vi "relayOpenCircuitTest.vi"() -> ()   [LabVIEW 2023]
panel:
  in  "switchTime/s":i32=50
  in  "relay 2 (unshort)":bool
  in  "flag 2":bool
  out "error out":errorcluster
  in  "relay 1 (open)":bool
  in  "flag 1":bool
  in  "error in (no error)":errorcluster
  in  "VISA relay":refnum<visa-resource-name>
  in  "VISA 2110 current":refnum<visa-resource-name>="USB0::0x05E6::0x2110::8017058::INSTR"
  in  "VISA 2110 voltage":refnum<visa-resource-name>="USB0::0x05E6::0x2110::8016020::INSTR"
  out "error out 4":errorcluster
  out "error out 3":errorcluster
  in  "stop 5":bool
  out "Current through 330 ohm resistor inner segment/mA 6":cluster{"Y":dbl[], "Y":dbl[]}[](graph)
  out "Voltage across 330 ohm resistor 7":dbl[](graph)
  out "Voltage across 330 ohm resistor 8":dbl[](array[numeric])
  out "Current time":timestamp
  out "Voltage/V":cluster{"Y":dbl[], "Y":dbl[]}[](graph)
  out "Voltage":dbl[](graph)
  out "Voltage":dbl[](array[numeric])
  in  "Filename 4":path caption="Filename"
  in  "Camera":bool=TRUE
  out "Start time":timestamp
  in  "Countdown/s":i32=3
  out "Timer":dbl
  in  "error in (no error) 3":errorcluster
  in  "error in (no error) 2":errorcluster
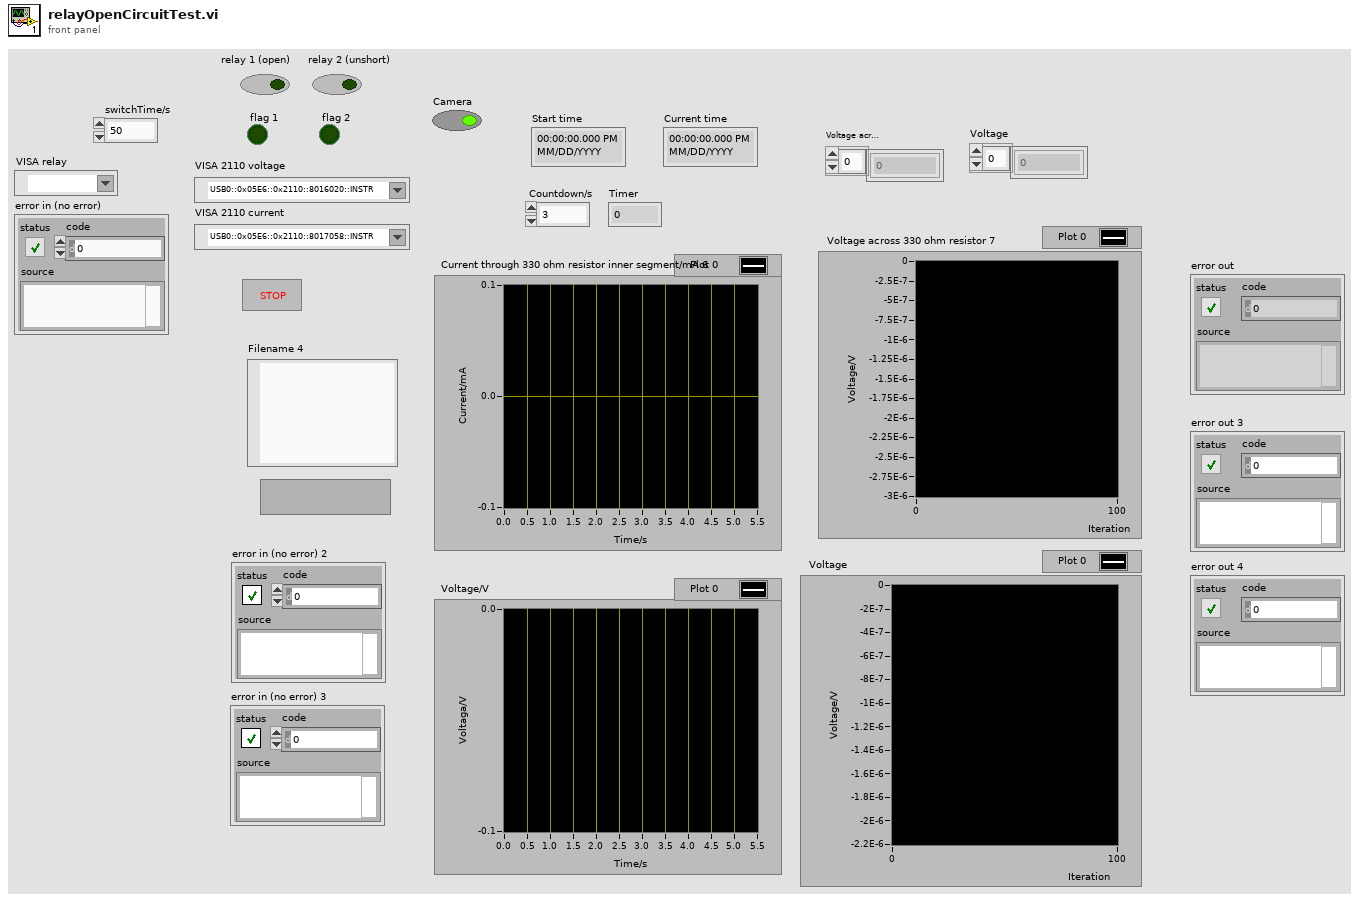
[diagram p1: front panel]
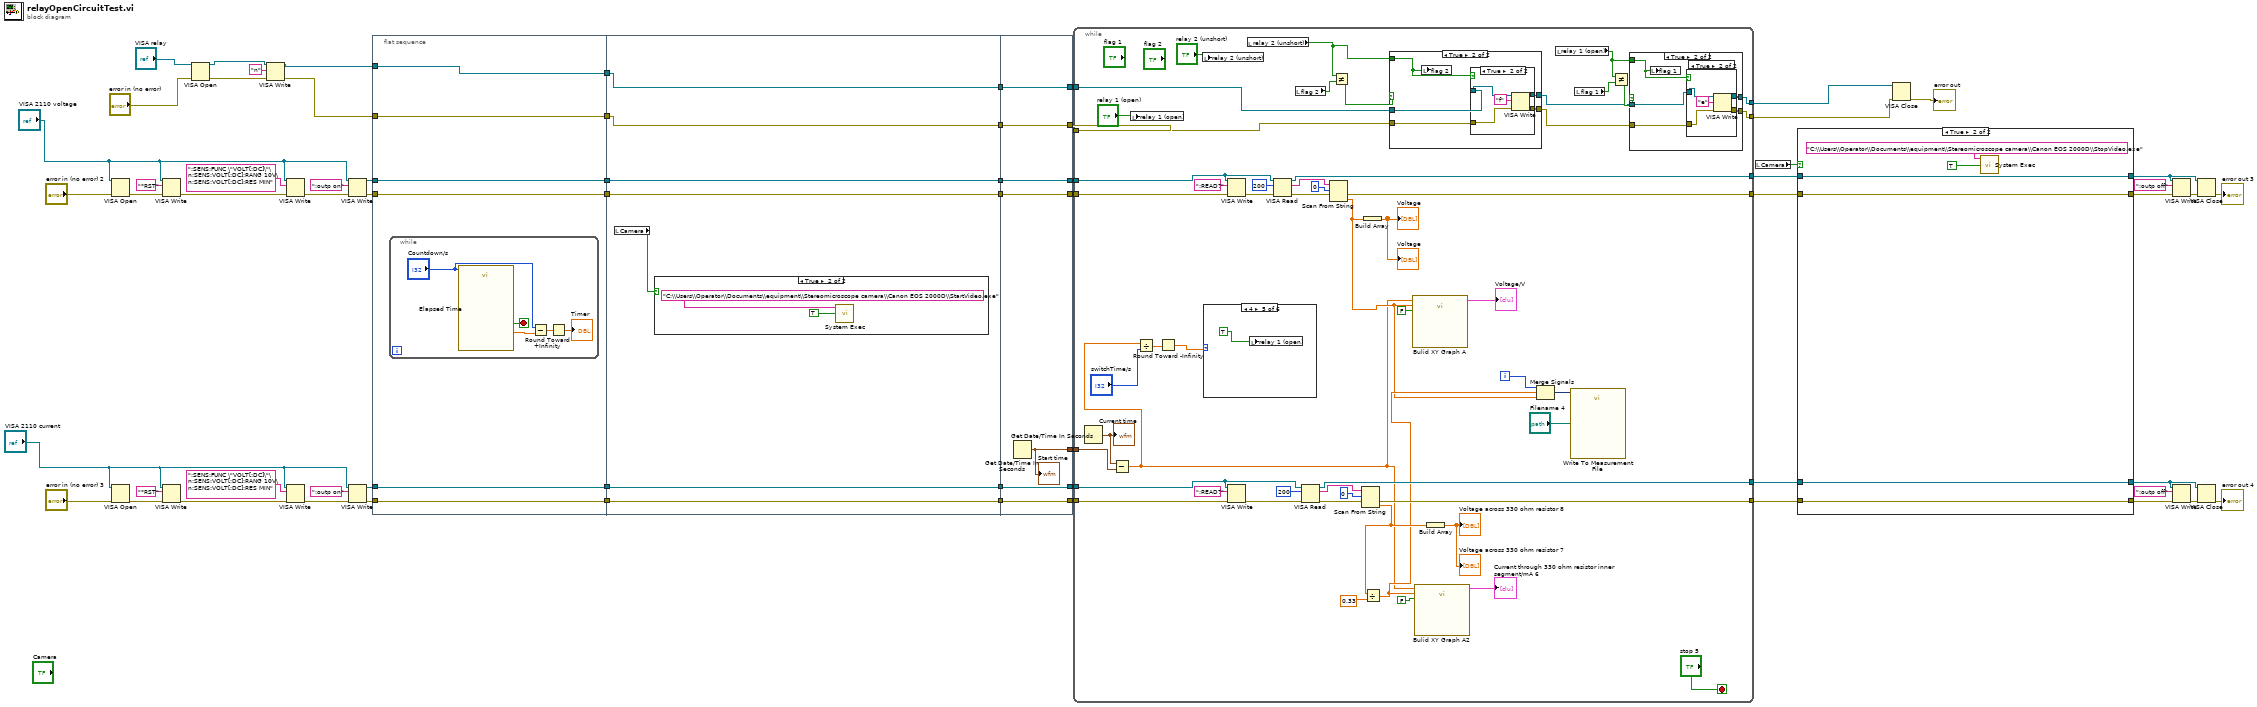
[diagram p0: block diagram]
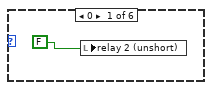
[diagram p3: hidden frame]
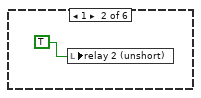
[diagram p4: hidden frame]
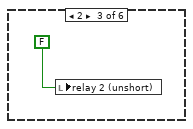
[diagram p5: hidden frame]
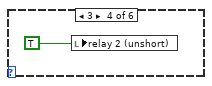
[diagram p6: hidden frame]
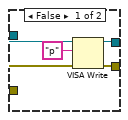
[diagram p9: hidden frame]
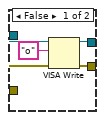
[diagram p11: hidden frame]
diagram:
  n1 = VISA Open(error in (no error)="error in (no error) 2", VISA resource name="VISA 2110 voltage") -> (error out=w64:errorcluster)  [unwired: 3 in, 1 out]
  n2 = VISA Open(error in (no error)="error in (no error) 3", VISA resource name="VISA 2110 current") -> (error out=w58:errorcluster)  [unwired: 3 in, 1 out]
  n3 = VISA Write(VISA resource name="VISA 2110 voltage", write buffer="*RST" ("数据"), error in (no error)=w64) -> (error out=w63:errorcluster)  [unwired: 2 out]
  n4 = VISA Write(VISA resource name="VISA 2110 current", write buffer="*RST" ("数据"), error in (no error)=w58) -> (error out=w57:errorcluster)  [unwired: 2 out]
  n5 = VISA Open(error in (no error)="error in (no error)", VISA resource name="VISA relay") -> (VISA resource name=w4:refnum<visa-resource-name>, error out=w3:errorcluster)  [unwired: 3 in]
  n6 = VISA Write(VISA resource name=w4, write buffer="n", error in (no error)=w3) -> (VISA resource name out=w1:refnum<visa-resource-name>, error out=w2:errorcluster)  [unwired: 1 out]
  n7 = VISA Write(VISA resource name="VISA 2110 voltage", write buffer=":SENS:FUNC \"VOLT[:DC]\"\n:SENS:VOLT[:DC]:RANG 10V\n:SENS:VOLT[:DC]:RES MIN" ("address string"), error in (no error)=w63) -> (error out=w62:errorcluster)  [unwired: 2 out]
  n8 = VISA Write(VISA resource name="VISA 2110 current", write buffer=":SENS:FUNC \"VOLT[:DC]\"\n:SENS:VOLT[:DC]:RANG 10V\n:SENS:VOLT[:DC]:RES MIN" ("address string"), error in (no error)=w57) -> (error out=w56:errorcluster)  [unwired: 2 out]
  n9 = VISA Write(VISA resource name="VISA 2110 voltage", write buffer=":outp on" ("数据"), error in (no error)=w62) -> (VISA resource name out=w42:refnum<visa-resource-name>, error out=w41:errorcluster)  [unwired: 1 out]
  n10 = VISA Write(VISA resource name="VISA 2110 current", write buffer=":outp on" ("数据"), error in (no error)=w56) -> (VISA resource name out=w40:refnum<visa-resource-name>, error out=w39:errorcluster)  [unwired: 1 out]
  n11 = flat-sequence {
    tunnel: w41 -> [w69]
    tunnel: w42 -> [w70]
    tunnel: [w70] -> w50
    tunnel: [w69] -> w49
    tunnel: w40 -> [w68]
    tunnel: [w68] -> w48
    tunnel: w39 -> [w67]
    tunnel: [w67] -> w47
    tunnel: [w66] -> w14
    tunnel: w1 -> [w66]
    tunnel: [w65] -> w11
    tunnel: w2 -> [w65]
    tunnel: w50 -> [w82]
    tunnel: w49 -> [w81]
    tunnel: [w82] -> w46
    tunnel: [w81] -> w45
    tunnel: [w79] -> w44
    tunnel: w48 -> [w79]
    tunnel: [w78] -> w43
    tunnel: w47 -> [w78]
    tunnel: w14 -> [w77]
    tunnel: [w77] -> w13
    tunnel: w11 -> [w76]
    tunnel: [w76] -> w10
    tunnel: [w89] -> w38
    tunnel: [w90] -> w36
    tunnel: [w91] -> w37
    tunnel: w46 -> [w91]
    tunnel: w45 -> [w90]
    tunnel: [w88] -> w35
    tunnel: w44 -> [w88]
    tunnel: [w87] -> w34
    tunnel: w43 -> [w87]
    tunnel: [w86] -> w12
    tunnel: w13 -> [w86]
    tunnel: [w85] -> w9
    tunnel: w10 -> [w85]
    frame #0 {
      n12 = while {
        stop <- w73 stop-if-true
        n13 = call "Elapsed Time"("Time Target (s)"="Countdown/s") -> ("Elapsed Time (s)"=w75:dbl, "Time has Elapsed"=w73:bool)  [unwired: 11 in, 6 out]
        n14 = Subtract(x="Countdown/s", y=w75) -> (x-y=w72:dbl)
        n15 = Round Toward +Infinity(x=w72) -> (ceil(x): smallest int >= x=→"Timer":dbl)
      }
    }
    frame #1 {
      n16 = local read "Camera"() -> (w80:bool)
      n17 = case shown="True" w80 {
        frame False {
        }
        frame True {
          n18 = call <vilib>:"System Exec.vi"("wait until completion? (T)"=TRUE, "command line"="C:\\Users\\Operator\\Documents\\equipment\\Stereomicroscope camera\\Canon EOS 2000D\\StartVideo.exe") -> ()  [unwired: 6 in, 4 out]
        }
      }
    }
    frame #2 {
      n19 = Get Date/Time In Seconds() -> (seconds since 1Jan1904=w89:timestamp)
      "Start time" <- w89
    }
  }
  n20 = while {
    tunnel: w38 -> [w145]
    tunnel: w37 -> [w144]
    tunnel: w36 -> [w143]
    tunnel: w35 -> [w142]
    tunnel: w34 -> [w141]
    tunnel: [w139] -> w26
    tunnel: [w138] -> w24
    tunnel: [w137] -> w22
    tunnel: [w136] -> w20
    tunnel: w12 -> [w125]
    tunnel: w9 -> [w128]
    tunnel: [w132] -> w8
    tunnel: [w131] -> w7
    i -> [w135]
    stop <- "stop 5" stop-if-true
    n21 = Get Date/Time In Seconds() -> (seconds since 1Jan1904=w107:timestamp)
    "Current time" <- w107
    n22 = Subtract(x=w107, y=w145) -> (x-y=w95:dbl)
    n23 = local write "relay 1 (open)"("relay 1 (open)") -> ()
    n24 = Divide(x=w95, y="switchTime/s") -> (x/y=w96:dbl)
    n25 = Round Toward -Infinity(1:w96) -> (0:w94:dbl)
    n26 = local write "relay 2 (unshort)"("relay 2 (unshort)") -> ()
    n27 = case shown="4" w94 {
      frame 0 {
        n28 = local write "relay 2 (unshort)"(FALSE) -> ()
      }
      frame 1 {
        n29 = local write "relay 2 (unshort)"(TRUE) -> ()
      }
      frame 2 {
        n30 = local write "relay 2 (unshort)"(FALSE) -> ()
      }
      frame 3 {
        n31 = local write "relay 2 (unshort)"(TRUE) -> ()
      }
      frame 4 {
        n32 = local write "relay 1 (open)"(TRUE) -> ()
      }
      frame 5, Default {
      }
    }
    n33 = VISA Write(VISA resource name=w144, write buffer=":READ?" ("数据"), error in (no error)=w143) -> (error out=w120:errorcluster)  [unwired: 2 out]
    n34 = VISA Write(VISA resource name=w142, write buffer=":READ?" ("数据"), error in (no error)=w141) -> (error out=w111:errorcluster)  [unwired: 2 out]
    n35 = local read "relay 2 (unshort)"() -> (w92:bool)
    n36 = VISA Read(VISA resource name=w144, byte count=200 ("字节总数"), error in (no error)=w120) -> (VISA resource name out=w139:refnum<visa-resource-name>, read buffer=w122:string, error out=w121:errorcluster)  [unwired: 1 out]
    n37 = local read "flag 2"() -> (w130:bool)
    n38 = VISA Read(VISA resource name=w142, byte count=200 ("字节总数"), error in (no error)=w111) -> (VISA resource name out=w137:refnum<visa-resource-name>, read buffer=w113:string, error out=w112:errorcluster)  [unwired: 1 out]
    n39 = Scan From String(input string=w122, initial scan location=u32 0 ("初始扫描位置"), error in=w121) -> (error out=w138:errorcluster, output 1=w100:dbl)  [unwired: 2 in, 2 out]
    n40 = Not Equal?(x=w92, y=w130) -> (x != y?=w129:bool)
    n41 = Scan From String(input string=w113, initial scan location=u32 0 ("初始扫描位置"), error in=w112) -> (error out=w136:errorcluster, output 1=w102:dbl)  [unwired: 2 in, 2 out]
    n42 = Build Array(w100) -> (→"Voltage" →"Voltage":dbl[])
    n43 = Divide(x=w102, y=0.33) -> (x/y=w101:dbl)
    n44 = case shown="True" w129 {
      tunnel: w92 -> [_ w157]
      tunnel: w128 -> [w152 w153]
      tunnel: [w151 w156] -> w127
      tunnel: [w152 w155] -> w126
      tunnel: w125 -> [w151 w154]
      frame False {
      }
      frame True {
        n45 = local write "flag 2"(w157) -> ()
        n46 = case shown="True" w157 {
          tunnel: w154 -> [w159 w167]
          tunnel: w153 -> [w158 w165]
          tunnel: [w161 w164] -> w156
          tunnel: [w160 w163] -> w155
          frame False {
            n47 = VISA Write(VISA resource name=w159, write buffer="p", error in (no error)=w158) -> (VISA resource name out=w161:refnum<visa-resource-name>, error out=w160:errorcluster)  [unwired: 1 out]
          }
          frame True {
            n48 = VISA Write(VISA resource name=w167, write buffer="f", error in (no error)=w165) -> (VISA resource name out=w164:refnum<visa-resource-name>, error out=w163:errorcluster)  [unwired: 1 out]
          }
        }
      }
    }
    n49 = call "Bulid XY Graph A"("Reset"=FALSE, "Y Input"=w100, "X Input"=w95) -> ("XY Graph"=→"Voltage/V":cluster{"X":dbl[], "Y":dbl[]}[])  [unwired: 7 in, 1 out]
    n50 = call "Bulid XY Graph A2"("Reset"=FALSE, "Y Input"=w101, "X Input"=w95) -> ("XY Graph"=→"Current through 330 ohm resistor inner segment/mA 6":cluster{"X":dbl[], "Y":dbl[]}[])  [unwired: 7 in, 1 out]
    n51 = Build Array(w102) -> (→"Voltage across 330 ohm resistor 8" →"Voltage across 330 ohm resistor 7":dbl[])
    n52 = Merge Signals(w135, w101, w100) -> (w124:dynamicdata)
    n53 = local read "relay 1 (open)"() -> (w98:bool)
    n54 = call "Write To Measurement File"("Signals"=w124, "Filename"="Filename 4") -> ()  [unwired: 15 in, 3 out]
    n55 = local read "flag 1"() -> (w134:bool)
    n56 = Not Equal?(x=w98, y=w134) -> (x != y?=w133:bool)
    n57 = case shown="True" w133 {
      tunnel: w98 -> [_ w174]
      tunnel: w126 -> [w169 w170]
      tunnel: [w168 w173] -> w132
      tunnel: [w169 w172] -> w131
      tunnel: w127 -> [w168 w171]
      frame False {
      }
      frame True {
        n58 = local write "flag 1"(w174) -> ()
        n59 = case shown="True" w174 {
          tunnel: w171 -> [w176 w184]
          tunnel: w170 -> [w175 w182]
          tunnel: [w178 w181] -> w173
          tunnel: [w177 w180] -> w172
          frame False {
            n60 = VISA Write(VISA resource name=w176, write buffer="o", error in (no error)=w175) -> (VISA resource name out=w178:refnum<visa-resource-name>, error out=w177:errorcluster)  [unwired: 1 out]
          }
          frame True {
            n61 = VISA Write(VISA resource name=w184, write buffer="e", error in (no error)=w182) -> (VISA resource name out=w181:refnum<visa-resource-name>, error out=w180:errorcluster)  [unwired: 1 out]
          }
        }
      }
    }
  }
  n62 = local read "Camera"() -> (w27:bool)
  n63 = case shown="True" w27 {
    tunnel: [w188 w192] -> w25
    tunnel: w26 -> [w188 w192]
    tunnel: [w187 w191] -> w23
    tunnel: w24 -> [w187 w191]
    tunnel: [w186 w190] -> w21
    tunnel: w22 -> [w186 w190]
    tunnel: [w185 w189] -> w19
    tunnel: w20 -> [w185 w189]
    frame False {
    }
    frame True {
      n64 = call <vilib>:"System Exec.vi"("wait until completion? (T)"=TRUE, "command line"="C:\\Users\\Operator\\Documents\\equipment\\Stereomicroscope camera\\Canon EOS 2000D\\StopVideo.exe") -> ()  [unwired: 6 in, 4 out]
    }
  }
  n65 = VISA Close(VISA resource name=w8, error in (no error)=w7) -> (error out=→"error out":errorcluster)
  n66 = VISA Write(VISA resource name=w25, write buffer=":outp off" ("数据"), error in (no error)=w23) -> (error out=w32:errorcluster)  [unwired: 2 out]
  n67 = VISA Write(VISA resource name=w21, write buffer=":outp off" ("数据"), error in (no error)=w19) -> (error out=w29:errorcluster)  [unwired: 2 out]
  n68 = VISA Close(VISA resource name=w25, error in (no error)=w32) -> (error out=→"error out 3":errorcluster)
  n69 = VISA Close(VISA resource name=w21, error in (no error)=w29) -> (error out=→"error out 4":errorcluster)
